vi "Write Reader IDs.vi"(8 "error in (no error)":errorcluster, 10 "reader IDs":string[](array[string]), 11 "Waveforms (N Ch) in":refnum<class "Waveforms (N Ch).lvclass">) -> (0 "error out":errorcluster, 3 "Waveforms (N Ch) out":refnum<class "Waveforms (N Ch).lvclass">)   [LabVIEW 2017, in "Waveforms (N Ch).lvclass"]
uses:
  <vilib>/addons/_NISVFA/_Shared subVIs/Data Objects/Waveforms (DBL)/Waveforms (N Ch).lvclass
  C:/Program Files (x86)/National Instruments/LabVIEW 2017/vi.lib/addons/_NISVFA/_Shared subVIs/Data Objects/Data/Data.lvclass
  <vilib>/Utility/error.llb/whitespace.ctl
  <vilib>/addons/_NISVFA/_Shared subVIs/Data Objects/Data/Data.lvclass/Data.ctl
  <vilib>/addons/_NISVFA/_Shared subVIs/Data Objects/Data/Data.lvclass
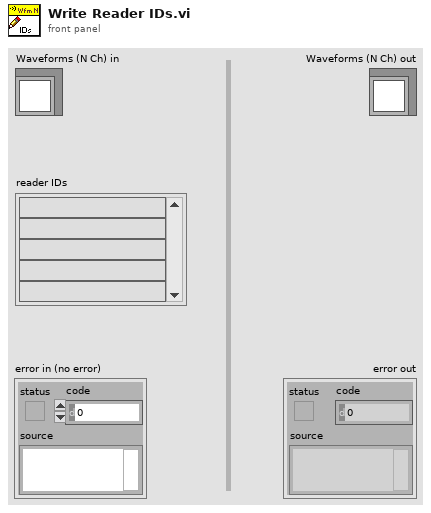
[diagram p1: front panel]
types:
  T1 = typedef "whitespace.ctl" = u16
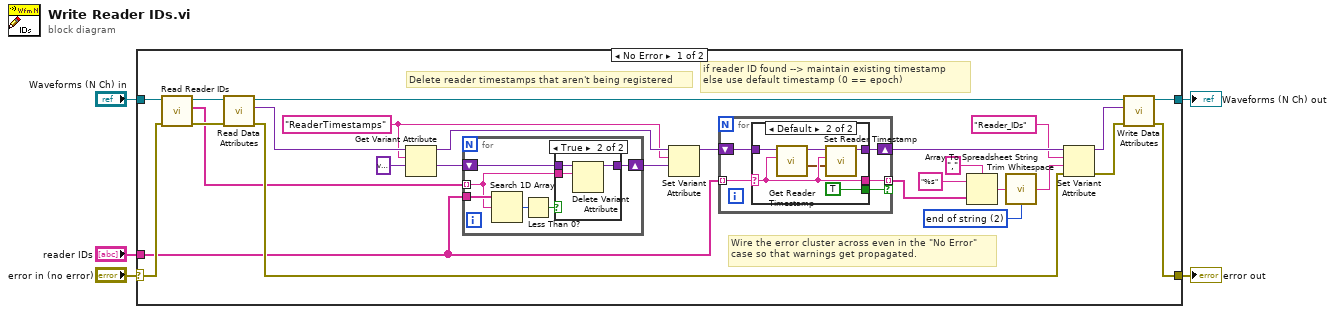
[diagram p0: block diagram]
diagram:
  n1 = case shown="No Error" "error in (no error)" {
    selector: "error in (no error)" -> [w15 w56]
    tunnel: [w21 w56] -> w4
    tunnel: [w24 w55] -> w2
    tunnel: "Waveforms (N Ch) in" -> [w20 w55]
    tunnel: "reader IDs" -> [w10 _]
    frame No Error {
      w6 = "ReaderTimestamps" ("name")
      w31 = T1 2 items=["both", "start of string", "end of string"] ("location (both)")
      # "if reader ID found --> maintain existing timestamp\nelse use default timestamp (0 == epoch)"
      # "Delete reader timestamps that aren't being registered"
      # "Wire the error cluster across even in the \"No Error\"\ncase so that warnings get propagated."
      n2 = call <vilib>:"Read Reader IDs.vi"("error in (no error)"=w15, "Waveforms (N Ch) in"=w20) -> ("error out"=w17:errorcluster, "reader IDs"=w14:string[], "Waveforms (N Ch) out"=w19:refnum<class "Waveforms (N Ch).lvclass">)  [unwired: 7 in]
      n3 = call <vilib>:"Read Data Attributes.vi"("error in (no error)"=w17, "Data in"=w19) -> ("error out"=w16:errorcluster, "data attributes"=w12:variant, "Data out"=w18:refnum<class "Waveforms (N Ch).lvclass">)  [unwired: 7 in]
      n4 = Get Variant Attribute(Variant=w12, name=w6, default value (empty Variant)=variant ("ReaderTimestamps")) -> (duplicate Variant=w7:variant, value=w11:variant)  [unwired: 1 in, 2 out]
      n5 = for {
        tunnel: w14 -> [w33] mode=indexing
        tunnel: w10 -> [w38]
        shift-right: [w36] -> w8
        shift-left: w11 -> [w35]
        n6 = Search 1D Array(1D array=w38, element=w33) -> (index of element=w37:i32)  [unwired: 1 in]
        n7 = Less Than 0?(x=w37) -> (x < 0?=w34:bool)
        n8 = case shown="True" w34 {
          tunnel: [w39 w42] -> w36
          tunnel: w35 -> [w39 w41]
          tunnel: w33 -> [_ w40]
          frame False {
          }
          frame True {
            n9 = Delete Variant Attribute(6:w40, 7:w41) -> (3:w42:variant)  [unwired: 1 in, 2 out]
          }
        }
      }
      n10 = Set Variant Attribute(Variant=w7, name=w6, value=w8) -> (Variant out=w9:variant)  [unwired: 1 in, 2 out]
      n11 = for {
        shift-right: [w46] -> w27
        shift-left: w9 -> [w47]
        tunnel: w10 -> [w45] mode=indexing
        tunnel: [w44] -> w28 mode=indexing if=w43
        n12 = case shown="Default" w45 {
          selector: w45 -> [_ w50]
          tunnel: w47 -> [w48 w52]
          tunnel: [w48 w54] -> w46
          tunnel: [_ w50] -> w44
          tunnel: [_ TRUE] -> w43
          frame "" {
          }
          frame Default {
            n13 = call <vilib>:"Get Reader Timestamp.vi"("ID"=w50, "data attributes"=w52) -> ("timestamp"=w49:timestamp, "data attributes"=w51:variant)  [unwired: 8 in]
            n14 = call <vilib>:"Set Reader Timestamp.vi"("timestamp"=w49, "ID"=w50, "data attributes in"=w51) -> ("data attributes out"=w54:variant)  [unwired: 8 in]
          }
        }
      }
      n15 = Array To Spreadsheet String(delimiter (Tab)=",", array=w28, 3:"%s" ("format string")) -> (spreadsheet string=w32:string)
      n16 = call <vilib>:"Trim Whitespace.vi"("string"=w32, "location (both)"=w31) -> ("trimmed string"=w25:string)
      n17 = Set Variant Attribute(Variant=w27, name="Reader_IDs", value=w25, error in=w16) -> (Variant out=w23:variant, error out=w22:errorcluster)  [unwired: 1 out]
      n18 = call <vilib>:"Write Data Attributes.vi"("error in (no error)"=w22, "data attributes"=w23, "Data in"=w18) -> ("error out"=w21:errorcluster, "Data out"=w24:refnum<class "Waveforms (N Ch).lvclass">)  [unwired: 7 in]
    }
    frame Error {
    }
  }
  "error out" <- w4
  "Waveforms (N Ch) out" <- w2
